vi "Reset Revolution Sensor Status (uSMC).vi"(3 "error in (no error)":errorcluster, 4 "Index":i32, 5 "Visa Array in":refnum<visa-resource-name>[](array[refnum])) -> (0 "error out":errorcluster, 2 "Visa Array out":refnum<visa-resource-name>[](array[refnum]))   [LabVIEW 2010, in "SignalWriterMH110203USBStepperMotor.lvclass"]
uses:
  SignalWriterMH110203USBStepperMotor.lvclass
  class_data.vi
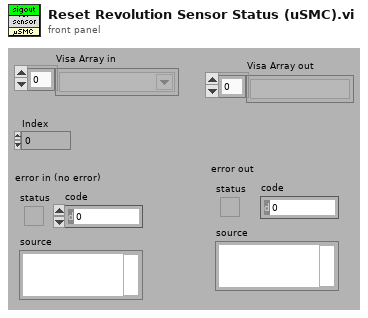
[diagram p1: front panel]
types:
  T1 = typedef "SignalWriterMH110203USBStepperMotor.lvclass/Mode Control (uSMC).ctl" = cluster{"Turn Buttons Off":bool, "Reduce Current":bool, "Power Off and Make a Whole Step":bool, "Emergency Power Off":bool, "Limit Switch 1 True State":bool, "Limit Switch 2 True State":bool, "Rotary Transducer TRUE State":bool, "Swap Limit Switches":bool, "Limit Switch 1 Operation Enabled":bool, "Limit Switch 2 Operation Enabled":bool, "Rotary Transducer Operation Enabled":bool, "Rotary Transducer Operation Select":bool, "Button 1 True State":bool, "Button 2 True State":bool, "Swap Buttons":bool, "Reset Rotary Transducer Check Positions":bool, "Output Syncronization Enabled":bool, "Reset Output Sync Count":bool, "Sync Operation":bool, "Sync Count":u32, "Power":bool, "Invert Sync Polarity":bool, "Use Encoder":bool, "Invert Encoder Direction":bool, "Reset Encoder To 0":bool, "Reset SM Enc Pos to Enc Pos":bool}
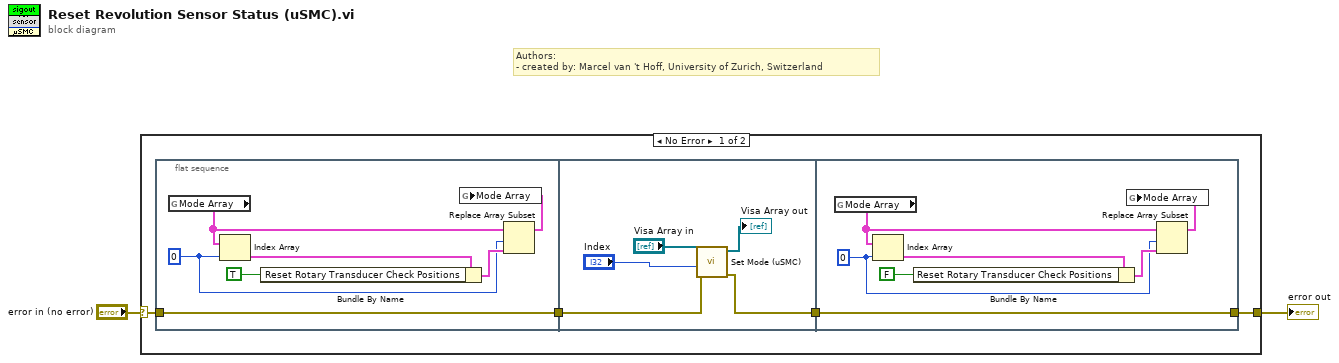
[diagram p0: block diagram]
diagram:
  # "Authors: \n- created by: Marcel van 't Hoff, University of Zurich, Switzerland"
  n1 = case shown="No Error" "error in (no error)" {
    selector: "error in (no error)" -> [w5 w26]
    tunnel: [w4 w26] -> w1
    frame No Error {
      n2 = flat-sequence {
        tunnel: [w7] -> w6
        tunnel: w5 -> [w7]
        tunnel: w6 -> [w15]
        tunnel: [w14] -> w3
        tunnel: [w19] -> w4
        tunnel: w3 -> [w19]
        frame #0 {
          w8 = 0 ("index")
          n3 = global read "class_data.vi" "Mode Array"() -> (w10:T1[])
          n4 = Index Array(array=w10, index=w8) -> (element=w13:T1)
          n5 = Bundle By Name(cluster=w13, "Reset Rotary Transducer Check Positions"=TRUE) -> (w11:T1)
          n6 = Replace Array Subset(array=w10, new element=w11, index=w8) -> (w9:T1[])
          n7 = global write "class_data.vi" "Mode Array"(w9) -> ()
        }
        frame #1 {
          n8 = call "Set Mode (uSMC).vi"("error in (no error)"=w15, "Index"="Index", "Visa Array in"="Visa Array in") -> ("error out"=w14:errorcluster, "Visa Array out"=→"Visa Array out":refnum<visa-resource-name>[])  [unwired: 7 in]
        }
        frame #2 {
          w20 = 0 ("index")
          n9 = global read "class_data.vi" "Mode Array"() -> (w22:T1[])
          n10 = Index Array(array=w22, index=w20) -> (element=w25:T1)
          n11 = Bundle By Name(cluster=w25, "Reset Rotary Transducer Check Positions"=FALSE) -> (w23:T1)
          n12 = Replace Array Subset(array=w22, new element=w23, index=w20) -> (w21:T1[])
          n13 = global write "class_data.vi" "Mode Array"(w21) -> ()
        }
      }
    }
    frame Error {
    }
  }
  "error out" <- w1
